vi "DFD FXP Simulation (I16).vi"(5 "input range":dbl=1.0, 7 "init? (T)":bool=TRUE, 8 "error in (no error)":errorcluster, 9 "filtering statistics in":T3(array[cluster])=[{"quantizer source"=0, "statistical information"={"max value"=-inf, "min value"=inf, "#overflows"=0, "#underflows"=0, "#operations"=0}}, {"quantizer source"=1, "statistical information"={"max value"=-inf, "min value"=inf, "#overflows"=0, "#underflows"=0, "#operations"=0}}, {"quantizer source"=2, "statistical information"={"max value"=-inf, "min value"=inf, "#overflows"=0, "#underflows"=0, "#operations"=0}}, {"quantizer source"=3, "statistical information"={"max value"=-inf, "min value"=inf, "#overflows"=0, "#underflows"=0, "#operations"=0}}, {"quantizer source"=4, "statistical information"={"max value"=-inf, "min value"=inf, "#overflows"=0, "#underflows"=0, "#operations"=0}}, {"quantizer source"=5, "statistical information"={"max value"=-inf, "min value"=inf, "#overflows"=0, "#underflows"=0, "#operations"=0}}, {"quantizer source"=6, "statistical information"={"max value"=-inf, "min value"=inf, "#overflows"=0, "#underflows"=0, "#operations"=0}}] {"statistical information"."min value" format="%.2f"; "statistical information"."max value" format="%.2f"; "quantizer source" items=["Coefficients a/k"=0, "Coefficients b/v"=7, "Input"=1, "Output"=2, "Multiplicand"=3, "Product"=4, "Sum"=5, "Delay"=6]}, 10 "filter in":T4={"mSRate_Fs"=1.0, "mSRate_Version"="2.0", "mSRate_Comments"="", "mSRate_OrgCoef"={"type"=enum."Undefined", "gain"=1.0, "coef a (k)"=[], "coef b (v)"=[]}, "mSRate_CurCoef"={"type"=enum."Undefined", "gain"=1.0, "coef a (k)"=[], "coef b (v)"=[]}, "mSRate_Quantized?"=FALSE, "mSRate_QCoef"={"type"=enum."Undefined", "gain"=1.0, "coef a (k)"=[], "coef b (v)"=[]}, "mSRate_QSettings"=[], "mSRate_Order"=0, "mSRate_Scaling"={"mSRate_ScaleByPowerOf2?"=FALSE, "mSRate_ScaleType"=enum."No Norm"}} {"mSRate_QSettings"."source" items=["Coef a/k"=0, "Coef b/v"=7, "Input"=1, "Output"=2, "Multiplicand"=3, "Product"=4, "Sum"=5, "Delay"=6, "Gain"=8]}, 11 "signal in":i16[](array[numeric])) -> (0 "error out":errorcluster, 1 "filtering statistics report":T3(array[cluster]) {"statistical information"."min value" format="%.2f"; "statistical information"."max value" format="%.2f"; "quantizer source" items=["Coefficients a/k"=0, "Coefficients b/v"=7, "Input"=1, "Output"=2, "Multiplicand"=3, "Product"=4, "Sum"=5, "Delay"=6]}, 2 "integer signal out":i32[](array[numeric]), 3 "DBL signal out":dbl[](array[numeric]) format="%.2f")   [LabVIEW 2017, in "NI_DigFilterLicensed.lvlib"]
doc: "Simulates the filtering process continuously and generates a filtering statistics report for a fixed-point filter. The data type you wire to the <B>signal in</B> input determines the polymorphic instance to use."
uses:
  <vilib>/addons/Digital Filter Design/NI_DigFilterLicensed.lvlib
  <vilib>/addons/Digital Filter Design/_Objects.llb/DFD Filter Obj.ctl
  <vilib>/addons/Digital Filter Design/_Objects.llb/DFD Filter Coef.ctl
  <vilib>/addons/Digital Filter Design/_Objects.llb/DFD Filter Structure Type Selector.ctl
  <vilib>/addons/Digital Filter Design/_Objects.llb/dfd_Internal Quantization Settings.ctl
  <vilib>/addons/Digital Filter Design/_Objects.llb/dfd_Internal Quantization Srcs.ctl
  <vilib>/addons/Digital Filter Design/_Objects.llb/DFD Coef Norm Type.ctl
  <vilib>/addons/Digital Filter Design/_Objects.llb/DFD Quantization Sources.ctl
  <vilib>/addons/Digital Filter Design/_Objects.llb/DFD FXP Statistics Data.ctl
  <vilib>/addons/Digital Filter Design/NI_DigFilter_FXP.lvlib
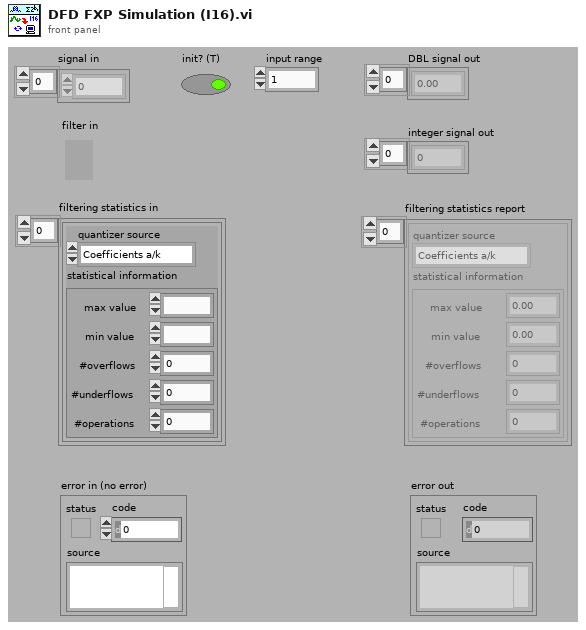
[diagram p1: front panel]
types:
  T1 = typedef "NI_DigFilterLicensed.lvlib/DFD Quantization Sources.ctl" = u16
  T2 = typedef "NI_DigFilterLicensed.lvlib/DFD FXP Statistics Data.ctl" = cluster{"max value":ext, "min value":ext, "#overflows":i32, "#underflows":i32, "#operations":i32}
  T3 = cluster{"quantizer source":T1, "statistical information":T2}[]
  T4 = typedef "NI_DigFilterLicensed.lvlib/DFD Filter Obj.ctl" = cluster{"mSRate_Fs":dbl, "mSRate_Version":string, "mSRate_Comments":string, "mSRate_OrgCoef":T5, "mSRate_CurCoef":T5, "mSRate_Quantized?":bool, "mSRate_QCoef":T5, "mSRate_QSettings":T7[], "mSRate_Order":i32, "mSRate_Scaling":cluster{"mSRate_ScaleByPowerOf2?":bool, "mSRate_ScaleType":T9}}
  T5 = typedef "NI_DigFilterLicensed.lvlib/DFD Filter Coef.ctl" = cluster{"type":T6, "gain":dbl, "coef a (k)":dbl[], "coef b (v)":dbl[]}
  T6 = typedef "NI_DigFilterLicensed.lvlib/DFD Filter Structure Type Selector.ctl" = enum16{"Undefined", "FIR Direct Form", "FIR Direct Form Transposed", "FIR Symmetric", "FIR Antisymmetric", "IIR Direct Form I", "IIR Direct Form I Transposed", "IIR Direct Form II", "IIR Direct Form II Transposed", "IIR Cascaded Second Order Sections Form I", "IIR Cascaded Second Order Sections Form I Transposed", "IIR Cascaded Second Order Sections Form II", "IIR Cascaded Second Order Sections Form II Transposed", "Lattice Allpass (basic sections)", "Lattice Allpass (one multiplier sections)", "Lattice Allpass (normalized sections)", "Lattice AR (basic sections)", "Lattice AR (one multiplier sections)", "Lattice AR (normalized sections)", "Lattice MA (minimum phase)", "Lattice MA (maximum phase)", "Lattice ARMA (basic sections)", "Lattice ARMA (one multiplier sections)", "Lattice ARMA (normalized sections)"}
  T7 = typedef "NI_DigFilterLicensed.lvlib/dfd_Internal Quantization Settings.ctl" = cluster{"source":T8, "wl":i16, "iwl":i16, "overflow mode":enum16{"Saturation", "Wrap"}, "rounding mode":enum16{"Nearest", "Truncation"}, "signed?":bool}
  T8 = typedef "NI_DigFilterLicensed.lvlib/dfd_Internal Quantization Srcs.ctl" = u16
  T9 = typedef "NI_DigFilterLicensed.lvlib/DFD Coef Norm Type.ctl" = enum16{"No Norm", "Time Domain 1-Norm", "Time Domain 2-Norm", "Time Domain Inf-Norm"}
  T10 = cluster{"Quantizer Source":T1, "statistics information":T2}[]
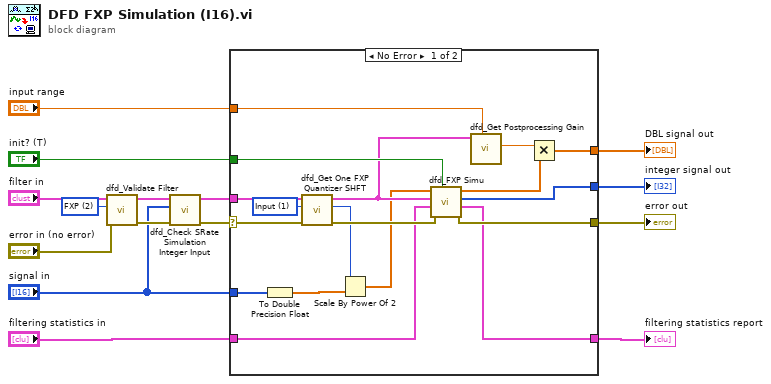
[diagram p0: block diagram]
diagram:
  w10 = u16 2 items=["Auto", "FLP Only", "FXP"] ("check option")
  n1 = call <vilib>:"dfd_Validate Filter.vi"("error in (no error)"="error in (no error)", "check option"=w10, "filter in"="filter in") -> ("error out"=w3:errorcluster, "filter out"=w8:T4)  [unwired: 7 out]
  n2 = call <vilib>:"dfd_Check SRate Simulation Integer Input.vi"("error in (no error)"=w3, "signal in"="signal in", "filter"=w8) -> ("error out"=w2:errorcluster, "dup multirate filter"=w4:T4)  [unwired: 7 out]
  n3 = case shown="No Error" w2 {
    selector: w2 -> [w26 w33]
    tunnel: "init? (T)" -> [w25 _]
    tunnel: [w32 w33] -> w14
    tunnel: "filtering statistics in" -> [w24 _]
    tunnel: [w31 _] -> w12
    tunnel: "signal in" -> [w30 _]
    tunnel: w4 -> [w21 _]
    tunnel: "input range" -> [w29 _]
    tunnel: [w27 _] -> w6
    tunnel: [w22 _] -> w5
    frame No Error {
      w19 = T8 1 items=["Coef a/k"=0, "Coef b/v"=7, "Input"=1, "Output"=2, "Multiplicand"=3, "Product"=4, "Sum"=5, "Delay"=6, "Gain"=8] ("quantization source")
      n4 = To Double Precision Float(number=w30) -> (double precision float=w18:dbl[])
      n5 = call <vilib>:"dfd_Get One FXP Quantizer SHFT.vi"("quantization source"=w19, "filter in"=w21) -> ("fwl SHFT"=w16:i16, "filter out"=w20:T4)  [unwired: 8 out]
      n6 = Scale By Power Of 2(n=w16, x=w18) -> (x*2^n=w17:dbl[])
      n7 = call <vilib>:"dfd_FXP Simu.vi"("init? (T)"=w25, "error in (no error)"=w26, "filtering statistics in"=w24, "filter"=w20, "signal in"=w17) -> ("error out"=w32:errorcluster, "filtering statistics out"=w31:T10, "integer signal out"=w22:i32[], "DBL signal out"=w28:dbl[])  [unwired: 2 in, 1 out]
      n8 = call <vilib>:"dfd_Get Postprocessing Gain.vi"("input range"=w29, "filter"=w20) -> ("DBL gain"=w23:dbl)  [unwired: 9 out]
      n9 = Multiply(x=w23, y=w28) -> (x*y=w27:dbl[])
    }
    frame Error {
    }
  }
  "DBL signal out" <- w6
  "error out" <- w14
  "filtering statistics report" <- w12
  "integer signal out" <- w5
